vi "QuickStartTemplate.vi"(11 "Error In":errorcluster) -> (15 "Error Out":errorcluster)   [LabVIEW 2016, in "Drona.lvlib"]
doc: "Template to start the initial steps for Drona Test"
uses:
  Drona.lvlib
  Stimulus/ControlValue/SetValueAuto.vi
  Assert/AssertControlValue/Equal.vi
  <vilib>/addons/_JKI Toolkits/Caraya/classes/Test/Test.lvclass
  Stimulus/ControlValue/ControlValue.lvlib
  Assert/AssertControlValue/AssertControlValue.lvlib
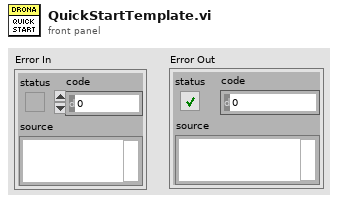
[diagram p1: front panel]
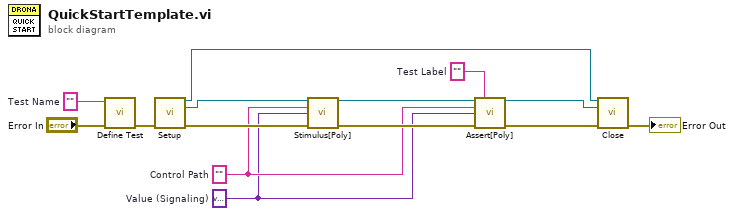
[diagram p0: block diagram]
diagram:
  w3 = ""  # Test Label
  w6 = variant  # Value (Signaling)
  w7 = ""  # Control Path
  w14 = ""  # Test Name
  n1 = call <vilib>:"Define Test.vi"("error in (no error)"="Error In", "Label (VI Title)"=w14) -> ("error out"=w12:errorcluster)  [unwired: 9 in]
  n2 = call "Setup.vi"("error in"=w12) -> ("Application Ref"=w2:refnum<vi>, "VI Reference Out"=w10:refnum<vi>, "error out"=w11:errorcluster)  [unwired: 12 in]
  n3 = call-poly "Stimulus[Poly].vi"("VI Reference In"=w10, "Control Path"=w7, "Value (Signaling)"=w6, "error in"=w11) -> ("VI Reference Out"=w8:refnum<vi>, "error out"=w9:errorcluster)  [unwired: 10 in]
  n4 = call-poly "Assert[Poly].vi"("VI Reference In"=w8, "Test Label"=w3, "Control Path"=w7, "Control Value"=w6, "Error In"=w9) -> ("VI Reference Out"=w4:refnum<vi>, "Error Out"=w5:errorcluster)  [unwired: 9 in]
  n5 = call "Close.vi"("Application Ref"=w2, "VI Reference"=w4, "error in"=w5) -> ("error out"=→"Error Out":errorcluster)  [unwired: 12 in]
